vi "AddLogMsg.vi"(7 "LogLevel":T1, 8 "Error":errorcluster[](array[cluster]), 10 "LogMessage":string) -> (0 "Error":errorcluster[](array[cluster]))   [LabVIEW 2014]
uses:
  LV_Config/Typedefs/eLogLvl.ctl
  LV_Config/Config.lvclass/Config.ctl
  LV_Config/Accessors/Read Logging.vi
  LV_Config/Config.lvclass
  <userlib>/NIST/NISTErrorLib/NISTErrorLib.lvlib
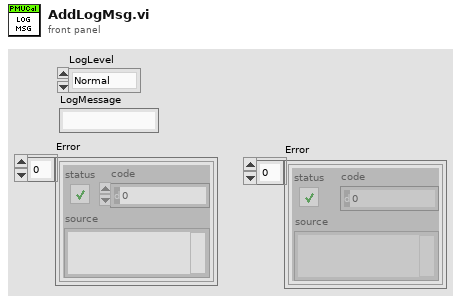
[diagram p1: front panel]
types:
  T1 = typedef "Config_class.lvlib/Config.lvclass/eLogLvl.ctl" = enum16{"Normal", "Verbose", "None"}
  T2 = typedef "Config_class.lvlib/Config.lvclass/Logging.ctl" = cluster{"eLogLvl":T1, "Log File Path":path, "btnLogFile":bool}
  T3 = enum16{"open", "replace", "create", "open or create", "replace or create", "replace or create with confirmation"}
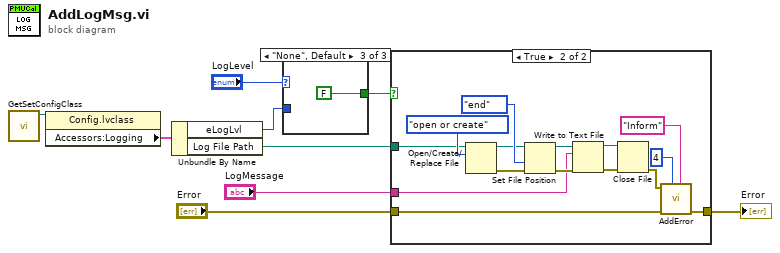
[diagram p0: block diagram]
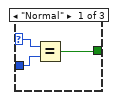
[diagram p3: hidden frame]
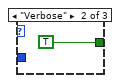
[diagram p4: hidden frame]
diagram:
  n1 = call "GetSetConfigClass.vi"() -> ("Ref out"=w9:refnum<class "Config.lvclass">)  [unwired: 11 in]
  n2 = property class="Config.lvclass"(reference=w9) -> ("Accessors:Logging"=w8:T2)  [unwired: 1 in, 2 out]
  n3 = Unbundle By Name(w8) -> ("eLogLvl"=w6:T1, "Log File Path"=w4:path)
  n4 = case shown="\"None\", Default" "LogLevel" {
    selector: "LogLevel" -> [w11 _ _]
    tunnel: [w10 TRUE FALSE] -> w5
    tunnel: w6 -> [w12 _ _]
    frame "Normal" {
      n5 = Equal?(x=w11, y=w12) -> (x = y?=w10:bool)
    }
    frame "Verbose" {
    }
    frame "None", Default {
    }
  }
  n6 = case shown="True" w5 {
    tunnel: w4 -> [_ w29]
    tunnel: "LogMessage" -> [_ w24]
    tunnel: [w15 w23] -> w2
    tunnel: "Error" -> [w15 w22]
    frame False {
    }
    frame True {
      n7 = Open/Create/Replace File(file path (use dialog)=w29, operation (0:open)=T3."open or create") -> (refnum out=w27:refnum<file>, error out=w16:errorcluster)  [unwired: 4 in, 1 out]
      n8 = Set File Position(refnum=w27, from (0:start)=enum16{"start", "end", "current"}."end", error in=w16) -> (refnum out=w26:refnum<file>, error out=w25:errorcluster)  [unwired: 1 in]
      n9 = Write to Text File(file (use dialog)=w26, text=w24, error in=w25) -> (refnum out=w20:refnum<file>, error out=w21:errorcluster)  [unwired: 1 in, 1 out]
      n10 = Close File(refnum=w20, error in=w21) -> (error out=w19:errorcluster)  [unwired: 1 out]
      n11 = call <userlib>:"AddError.vi"("Severity"="Inform", "Priority"=u8 4, "ErrorArray"=w22, "error in (no error)"=w19) -> ("ErrorArray"=w23:errorcluster[])  [unwired: 6 in, 1 out]
    }
  }
  "Error" <- w2
